vi "Live Display of Image and Spots.vi"(7 "Draw spots":bool, 8 "error in (no error)":errorcluster, 11 "img dst":refnum<image>=refnum) -> (0 "error out":errorcluster, 2 "Frame Duration":i64=66176, 3 "img out":refnum<image>)   [LabVIEW 2020]
uses:
  _Controls/Timer actions.ctl
  _Globals/pDataBuffer.vi
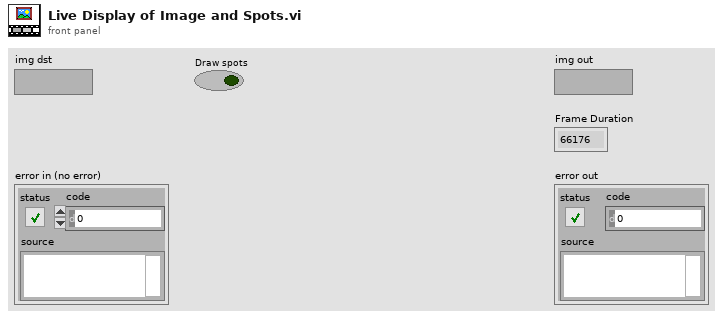
[diagram p1: front panel]
types:
  T1 = typedef "Timer actions.ctl" = enum16{"Reset", "Snap", "Total"}
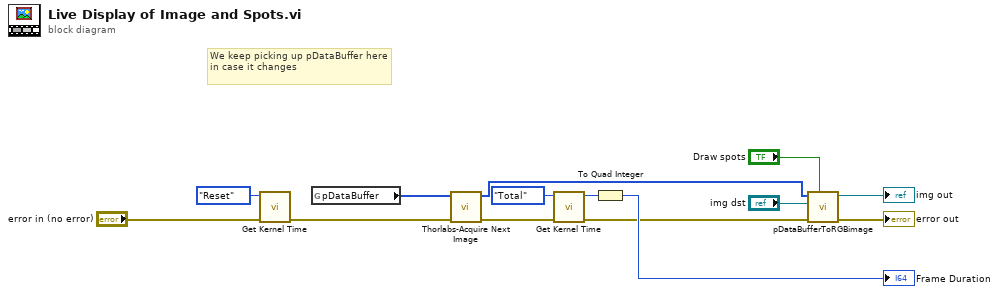
[diagram p0: block diagram]
diagram:
  # "We keep picking up pDataBuffer here in case it changes"
  n1 = call "Get Kernel Time.vi"("error in (no error) in"="error in (no error)", "Action (Snap)"=Timer_actions."Reset") -> ("error out"=w4:errorcluster)  [unwired: 8 in, 1 out]
  n2 = global read "pDataBuffer.vi" "pDataBuffer"() -> (w2:u16[])
  n3 = call "Thorlabs-Acquire Next Image.vi"("error in (no error)"=w4, "pDataBuffer in"=w2) -> ("error out"=w7:errorcluster, "pDataBuffer out"=w1:u16[])  [unwired: 7 in, 1 out]
  n4 = call "Get Kernel Time.vi"("error in (no error) in"=w7, "Action (Snap)"=Timer_actions."Total") -> ("error out"=w6:errorcluster, "Microseconds"=w10:u64)  [unwired: 8 in]
  n5 = To Quad Integer(1:w10) -> (0:→"Frame Duration":i64)
  n6 = call "pDataBufferToRGBimage.vi"("Draw spots"="Draw spots", "error in (no error)"=w6, "Img Dst"="img dst", "pDataBuffer"=w1) -> ("error out"=→"error out":errorcluster, "Img Out"=→"img out":refnum<image>)  [unwired: 6 in]
